vi "Main - Stop All Running Machine Base on TestType (SubVI).vi"(8 "error in (no error)":errorcluster, 11 "Cluster":T1 {"M Event" items=["Stop", "Running", "PID", "Up Limit", "Down Limit", "Load Limit"]; "Test Type" items=["Please Select", "Triaxial Shear", "Triaxial UU", "Shearbox", "Permeability", "Consolidation (Stepped Loading)/Swelling", "Saturation (Incremental)", "User Defined", "UCT", "Isotropic Consolidation", "Swelling Pressure"]; "Data"."Test Type" items=["Please Select", "Triaxial Shear", "Triaxial UU", "Shearbox", "Permeability", "Consolidation (Stepped Loading)/Swelling", "Saturation (Incremental)", "User Defined", "UCT", "Isotropic Consolidation", "Swelling Pressure"]}) -> (0 "error out":errorcluster)   [LabVIEW 2019]
uses:
  Controls/RunTest - Data Structure.ctl
  Controls/Test Panel - Data Structure.ctl
  Controls/Station - Test Type.ctl
  <vilib>/Utility/miscctls.llb/LVRowAndColumnTypeDef.ctl
  Controls/RunTest - Calculate Data.ctl
  <vilib>/httpClient/ClientHandle.ctl
  Controls/RunTest - Start Condition.ctl
  Controls/RunTest - Stop Condition.ctl
  Controls/UDP - Event.ctl
  Controls/UDP - Command.ctl
  <vilib>/httpClient/LabVIEWHTTPClient.lvlib
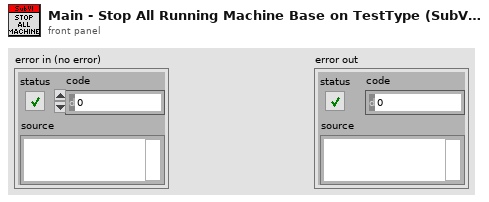
[diagram p1: front panel]
types:
  T1 = typedef "RunTest - Data Structure.ctl" = cluster{"Test Plan":string[], "PlanRow":i32, "Device Name":string[], "Timeout":i32, "Start?":bool, "Pause?":bool, "IP Address":string[], "LogRow":i32, "Logtype":u16, "Log Elapse":sgl, "Data":T2, "Stop log?":bool, "tdms":refnum<k34>, "Sensor Data":sgl[], "Start time":timestamp, "Prev Log Elapse":u32, "Plot":u16, "X-Axis":u16[], "Y-Axis":u16[], "XY":cluster{"X":dbl, "Y":dbl}[][], "End Stage?":bool, "1run":bool, "Condition":u16[], "Start Con":bool, "Log Con":bool, "Stop Con":bool, "Start Elapse":dbl, "Start Load":dbl, "Motor":i32, "StartRow":i32, "number log":i32, "Dir":bool, "Start time test":timestamp, "Auto":bool, "Check return?":bool, "Inv":cluster{"M":i32[], "Bool":bool[]}, "tdms temp":refnum<k34>, "Zero?":bool, "Plot Timer":dbl, "1st Run":bool, "TDMS Path":path, "MaxLoad":dbl, "Log Timer":sgl[], "Test Type":T3, "Log Sensor":string[], "Save?":bool, "1st Log":bool, "Y-Axis 2":u16[], "On Y-Axis 2":bool, "Decimal":u8[], "Init":cluster{"PWP TS":sgl, "Load TS":sgl, "Volume TS":sgl, "Disp TS":sgl, "CP":sgl, "Vol In":sgl, "Vol Out":sgl, "Load UCT":sgl, "Disp UCT":sgl, "PWP Sat":sgl, "CP Sat":sgl, "Volume IsoCons":sgl, "PWP IsoCons":sgl, "PWP TUU":sgl, "Load TUU":sgl, "Volume TUU":sgl, "Disp TUU":sgl, "Load Cons":sgl, "Disp Cons":sgl, "Volume Sat":sgl, "Vertical Load SB":sgl, "Vertical Disp SB":sgl, "H Disp SB":sgl, "H Load SB":sgl}, "Calc":T5, "Device Index":i32[], "Channel Index":i32[], "http ref":T6, "fileid":string, "Step Cons":cluster{"V Stress":sgl, "H Settlement":sgl}, "RunTest":bool, "Graph Last":i32, "Init?":bool, "Datalog":bool[], "Start":T7, "Stop":T8, "Running?":bool, "StartTime":dbl, "Log Prev Time":dbl, "KeyName":string[], "Test RunTime":dbl, "Log Prev Axial":dbl, "M Event":T9[], "Last Log":bool, "popup":bool, "PreStart UU":bool, "PreStart Sat":bool}
  T2 = typedef "Test Panel - Data Structure.ctl" = cluster{"Station":string, "Sample ID":string, "Job No":string, "Job Description":string, "Filename":string, "Test Type":T3, "Speciment No":string, "Depth":string, "Height":string, "Diameter/Length":string, "Weight":string, "Test Parameter":string, "Station[]":string[], "Edit Pos":T4, "Edit Pos Prev":T4, "Area":string, "Path":string}
  T3 = typedef "Station - Test Type.ctl" = u16
  T4 = typedef "LVRowAndColumnTypeDef.ctl" = cluster{"Row":i32, "Column":i32}
  T5 = typedef "RunTest - Calculate Data.ctl" = cluster{"TS":cluster{"Change PWP":sgl, "Change Vol":sgl, "Axial Load":sgl, "CiL":sgl, "Deviator":sgl, "Axial Strain":sgl, "MaxDeviator":sgl}, "TUU":cluster{"Change PWP":sgl, "Axial Load":sgl, "CiL":sgl, "Deviator":sgl, "Axial Strain":sgl, "MaxDeviator":sgl}, "Sat":cluster{"B Value":sgl, "PWP Diss":sgl, "CPP":sgl, "CV":sgl}, "Per":cluster{"Change Vol In":sgl, "Change Vol Out":sgl, "Mean Vol":sgl, "Gradient Pressure":sgl, "Outlet Flow":sgl, "Inlet Flow":sgl, "I X1":sgl, "I X2":sgl, "I Y1":sgl, "I Y2":sgl, "O X1":sgl, "O X2":sgl, "O Y1":sgl, "O Y2":sgl}, "Step Cons":cluster{"V Stress":sgl, "H Settlement":sgl, "Total H Settle":sgl, "Prev Total H":sgl}, "UCT":cluster{"ALC":sgl, "H Change":sgl, "Deviator":sgl, "Axial Strain":sgl, "V Stress":sgl, "MaxDeviator":sgl}, "ISO Cons":cluster{"CPP":sgl, "PWP Diss":sgl, "CV":sgl}, "SB":cluster{"Speci LenC":sgl, "Shear Strain":sgl, "H LC":sgl, "Normal Stress":sgl, "Shear Stress":sgl, "MaxShear":sgl}}
  T6 = typedef "LabVIEWHTTPClient.lvlib/ClientHandle.ctl" = refnum<k1>
  T7 = typedef "RunTest - Start Condition.ctl" = cluster{"Cons":cluster{"VS":dbl, "Delay":bool, "No Delay":dbl}, "Sat":cluster{"CP":dbl, "BP":dbl, "StartBP":bool, "Target CP":bool, "Target BP":bool}, "Iso":cluster{"Select":dbl, "BP":dbl, "IC2":dbl, "IC3":dbl, "IC4":dbl, ". IC6":bool, "IC6":dbl, "IC6-2":dbl, "Target":bool, "Time Cond":dbl, "Last PWP":dbl}, "TS":cluster{"SS":dbl, "Engage":bool, "ES":dbl, "LC":dbl, "PreStart":bool, "Trig SS":bool, "Drain":dbl}, "TUU":cluster{"SS":dbl, "Engage":bool, "ES":dbl, "LC":dbl, "PreStart":bool, "Trig SS":bool, "CP":dbl, "Delay Value":dbl, "Delay":bool, "CP PID":bool}, "UCT":cluster{"SS":dbl, "Engage":bool, "ES":dbl, "LC":dbl, "PreStart":bool, "Trig SS":bool}, "Enable?":bool, "SB":cluster{"SS":dbl, "Engage":bool, "ES":dbl, "LC":dbl, "PreStart":bool, "Trig SS":bool, "VS":dbl, "Delay Value":dbl, "Delay":bool, "VS PID":bool}, "Perm":cluster{"DP":dbl}}
  T8 = typedef "RunTest - Stop Condition.ctl" = cluster{"Cons":cluster{"Select":i32, "Disp":dbl, "Time":dbl, "Time2":dbl, "Disp 2":dbl, "Time Cond":dbl, "Last Disp":dbl, "Swell":bool}, "Sat":cluster{"Select":i32, "PP":dbl, "Time":dbl, "VC":dbl, "Time2":dbl, "Time Cond":dbl, "Last PP":dbl, ".B":bool, "B":dbl, "Last Vc":dbl, "Time Cond 2":dbl, "Time3":dbl, "Time Cond 3":dbl, "B Achieve":bool}, "Iso":cluster{"PP":dbl, "Time":dbl, "VC":dbl, "Time2":dbl, "Time Cond":dbl, "Last Vc":dbl, ".PP":bool, "Time Cond 2":dbl, "Select":i32}, "TS":cluster{"Axial":dbl, ".MaxDev":bool, "MaxDev Value":dbl, "Return":bool, "Reset":bool, "Prev Time":dbl, "PostStop Run":bool, "CP Stop":bool, "BP Stop":bool, "PostStop Trig":bool, "Reset Value":dbl, "BPTrig":bool, "CPTrig":bool, "VLCTrig":bool}, "TUU":cluster{"Axial":dbl, ".MaxDev":bool, "MaxDev Value":dbl, "Return":bool, "Reset":bool, "Prev Time":dbl, "PostStop Run":bool, "CP Stop":bool, "BP Stop":bool, "PostStop Trig":bool, "Reset Value":dbl, "BPTrig":bool, "CPTrig":bool, "VLCTrig":bool}, "UCT":cluster{"Axial":dbl, ".MaxDev":bool, "MaxDev Value":dbl, "Return":bool, "Reset":bool, "Prev Time":dbl, "PostStop Run":bool, "CP Stop":bool, "BP Stop":bool, "PostStop Trig":bool}, "Enable?":bool, "SB":cluster{"Shear":dbl, ".MaxShear":bool, "MaxShear Value":dbl, "Return":bool, "Reset":bool, "Prev Time":dbl, "PostStop Run":bool, "CP Stop":bool, "BP Stop":bool, "PostStop Trig":bool, "Reset Value":dbl, "BPTrig":bool, "CPTrig":bool, "VLCTrig":bool}, "Perm":cluster{"Max Time":bool, "Reset":bool, "PostStop Run":bool, "Ratio":bool, "Reset Value":dbl, "Time":dbl, "RatioTime":dbl, "RatioMore":dbl, "RatioLess":dbl, "Time Cond":dbl, "Time Cond 2":dbl, "Prev IF":dbl, "Prev OF":dbl, "PostStop Trig":bool, "BP Trig":bool, "DP Stop":bool, "BP Stop":bool, "CP Stop":bool, "CP Trig":bool}, "SP":cluster{".Max Time":bool, ".Time":bool, "Time":dbl, "MaxTime":dbl, "Time Cond":dbl, "Max Time Cond":dbl, "Stress":dbl}}
  T9 = typedef "UDP - Event.ctl" = u16
  T10 = cluster{"Station Name":string, "Key Value":string[], "Key Names":string[]}[]
  T11 = cluster{"Station Name":string, "Key Value":string[], "Key Names":string[]}
  T12 = typedef "UDP - Command.ctl" = enum16{"Stop", "Jog Up", "Jog Down", "Ramp Up", "Ramp Down", "PID Target", "PID Ramp", "Disp Run", "Read Ch Data", "Zero Channel", "Zero Disp", "Read Sensor", "Write Sensor", "Read ADC", "Write ADC", "Read PID", "Write PID", "Read Test", "Write Test", "Read System", "Write System", "Read Datalog", "Read Datalog Sensor"}
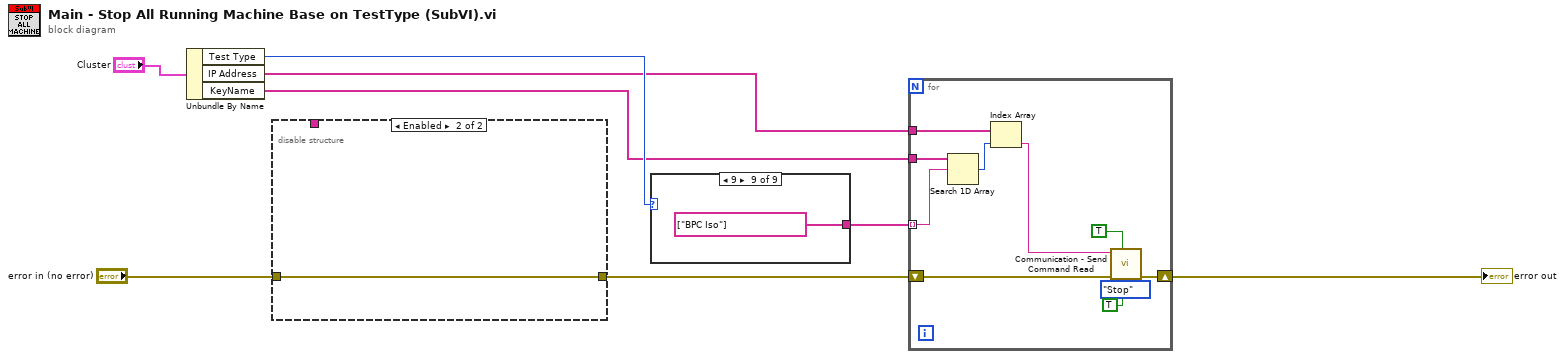
[diagram p0: block diagram]
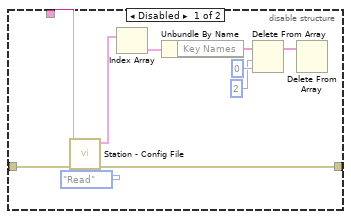
[diagram p2: hidden frame]
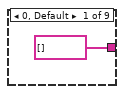
[diagram p3: hidden frame]
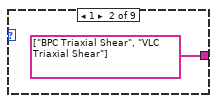
[diagram p4: hidden frame]
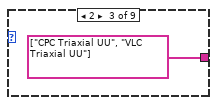
[diagram p5: hidden frame]
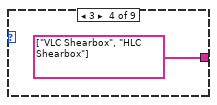
[diagram p6: hidden frame]
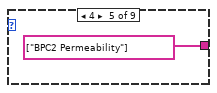
[diagram p7: hidden frame]
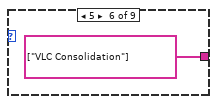
[diagram p8: hidden frame]
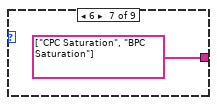
[diagram p9: hidden frame]
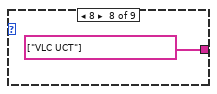
[diagram p10: hidden frame]
diagram:
  n1 = Unbundle By Name("Cluster") -> ("Test Type"=w7:T3, "IP Address"=w1:string[], "KeyName"=w2:string[])
  n2 = disable-structure shown="Enabled" {
    disable-tunnel: [w18 w19] -> w5
    disable-tunnel: _ -> [w17 _]
    disable-tunnel: "error in (no error)" -> [w16 w19]
    frame Disabled {
      n3 = call "Station - Config File.vi"("Action"=enum16{"Write", "Read", "Read All", "Remove"}."Read", "error in (no error)"=w16, "Station Name"=w17) -> ("error out"=w18:errorcluster, "Value Out"=w11:T10)  [unwired: 7 in]
      n4 = Index Array(array=w11) -> (element=w9:T11)  [unwired: 1 in]
      n5 = Unbundle By Name(w9) -> ("Key Names"=w14:string[])
      n6 = Delete From Array(array=w14, length=2, index=0) -> (array with subset deleted=w15:string[])  [unwired: 1 out]
      n7 = Delete From Array(array=w15) -> ()  [unwired: 2 in, 2 out]
    }
    frame Enabled {
    }
  }
  n8 = case shown="9" w7 {
    tunnel: [string[] [] string[] ["BPC Triaxial Shear", "VLC Triaxial Shear"] string[] ["CPC Triaxial UU", "VLC Triaxial UU"] string[] ["VLC Shearbox", "HLC Shearbox"] string[] ["BPC2 Permeability"] string[] ["VLC Consolidation"] string[] ["CPC Saturation", "BPC Saturation"] string[] ["VLC UCT"] string[] ["BPC Iso"]] -> w8
    frame 0, Default {
    }
    frame 1 {
    }
    frame 2 {
    }
    frame 3 {
    }
    frame 4 {
    }
    frame 5 {
    }
    frame 6 {
    }
    frame 8 {
    }
    frame 9 {
    }
  }
  n9 = for {
    tunnel: w2 -> [w38]
    shift-right: [w32] -> w6
    shift-left: w5 -> [w33]
    tunnel: w8 -> [w30] mode=indexing
    tunnel: w1 -> [w29]
    n10 = Search 1D Array(1D array=w38, element=w30) -> (index of element=w37:i32)  [unwired: 1 in]
    n11 = Index Array(array=w29, index=w37) -> (element=w31:string)
    n12 = call "Communication - Send Command Read.vi"("Fron?"=TRUE, "Bypass?"=TRUE, "error in (no error)"=w33, "Action"=UDP_-_Command."Stop", "Device IP Address"=w31) -> ("error out"=w32:errorcluster)  [unwired: 6 in]
  }
  "error out" <- w6
